vi "Host_FastOsziTest.vi"() -> ()   [LabVIEW 2012]
uses:
  <vilib>/Analysis/baseanly.llb/Mean (DBL).vi
  <vilib>/FPGAPlugInAG/PXIe-7962R/niLvFpga_Open_PXIe-7962R.vi
  <vilib>/rvi/interface/common/dynamic/niFpgaDynamicAddResources.vi
  <vilib>/Utility/error.llb/Error Cluster From Error Code.vi
  <vilib>/rvi/errors/niLvFpgaAdjustHostInterfaceError.vi
  <vilib>/FPGAPlugInAG/Dynamic/niLvFpga_Close_Dynamic.vi
  <vilib>/rvi/interface/nirviOpenFPGA/nirviOpenFPGA.xnode
  FPGA Bitfiles/NiFpga_AnalogDemultiplexerV2_NI5771.lvbitx
  <vilib>/rvi/interface/nirviReadWriteControl/nirviReadWriteControl.xnode
  <vilib>/rvi/interface/nirviMethod/nirviMethod.xnode
  <vilib>/rvi/interface/nirviCloseFPGA/nirviCloseFPGA.xnode
  <vilib>/rvi/interface/Simulation/niFpgaSimulationCallBeginRW.vi
  <vilib>/FPGAPlugInAG/Dynamic/niLvFpga_ReadFifo_Dynamic.vi
  <vilib>/rvi/errors/niLvFpgaMergeErrorWithErrorCode.vi
  <vilib>/Analysis/NI_AALPro.lvlib
  <vilib>/Analysis/NI_AALBase.lvlib
  NiFpgaLv.dll
panel:
  out "NOT Crosstalk":dbl format="%0.2f"
  out "Crosstalk":dbl format="%0.2f"
  in  "Save?":bool
  out "time to draw(ms) 2":i32=1000
  out "Area 1":picture
  in  "stop 2":bool
  in  "sized scatter plot cosmetics 2":T1={"min size"=1, "max size"=5, "maps to max size"=5, "color array"=[16711680, 65280, 255, 16776960, 16737792, 65535]}
  in  "cartesian axis attributes 2":T2={"x minimum"=1.0, "x maximum"=500.0, "x log?"=FALSE, "x precision"=1, "x format"=enum."Decimal", "y minimum"=60.0, "y maximum"=740.0, "y log?"=FALSE, "y precision"=1, "y format"=enum."Decimal"} {"x minimum" format="%0.2f"; "x maximum" format="%0.2f"; "y minimum" format="%0.2f"; "y maximum" format="%0.2f"}
  in  "?":u16(ring)=4 items=["Points", "Squares", "Circles", "Sized Squares", "Sized-Colored Squares", "Min-Max Lines"]
  in  "line color 2":u32(colorbox)=39168
  in  "text color 2":u32(colorbox)=65280
  in  "plot color 2":u32(colorbox)=16776960
  out "time to draw(ms)":i32=1000
  out "Area 2":picture
  in  "stop":bool
  in  "sized scatter plot cosmetics":T1={"min size"=1, "max size"=5, "maps to max size"=5, "color array"=[16711680, 65280, 255, 16776960, 16737792, 65535]}
  in  "cartesian axis attributes":T2={"x minimum"=1.0, "x maximum"=500.0, "x log?"=FALSE, "x precision"=1, "x format"=enum."Decimal", "y minimum"=60.0, "y maximum"=740.0, "y log?"=FALSE, "y precision"=1, "y format"=enum."Decimal"} {"x minimum" format="%0.2f"; "x maximum" format="%0.2f"; "y minimum" format="%0.2f"; "y maximum" format="%0.2f"}
  in  "?":u16(ring)=4 items=["Points", "Squares", "Circles", "Sized Squares", "Sized-Colored Squares", "Min-Max Lines"]
  in  "line color":u32(colorbox)=39168
  in  "text color":u32(colorbox)=65280
  in  "plot color":u32(colorbox)=16776960
  out "PMT histogram":T3(graph)
  out "Mean NOT pulse length":dbl format="%0.2f"
  out "Mean pulse length":dbl format="%0.2f"
  out "NOT Laser pulse length histogram":T3(graph)
  out "Laser pulse length histogram":T3(graph)
  out "Laser (Trigger In)":i16[](graph)
  in  "Samples per pixel":u32=10000
  out "IO Module\\AI Over Range":bool
  out "PMT (AI 0)":u8[](graph)
  # "Sampling at 1.5GHz => 0.66 ns sampling interval"
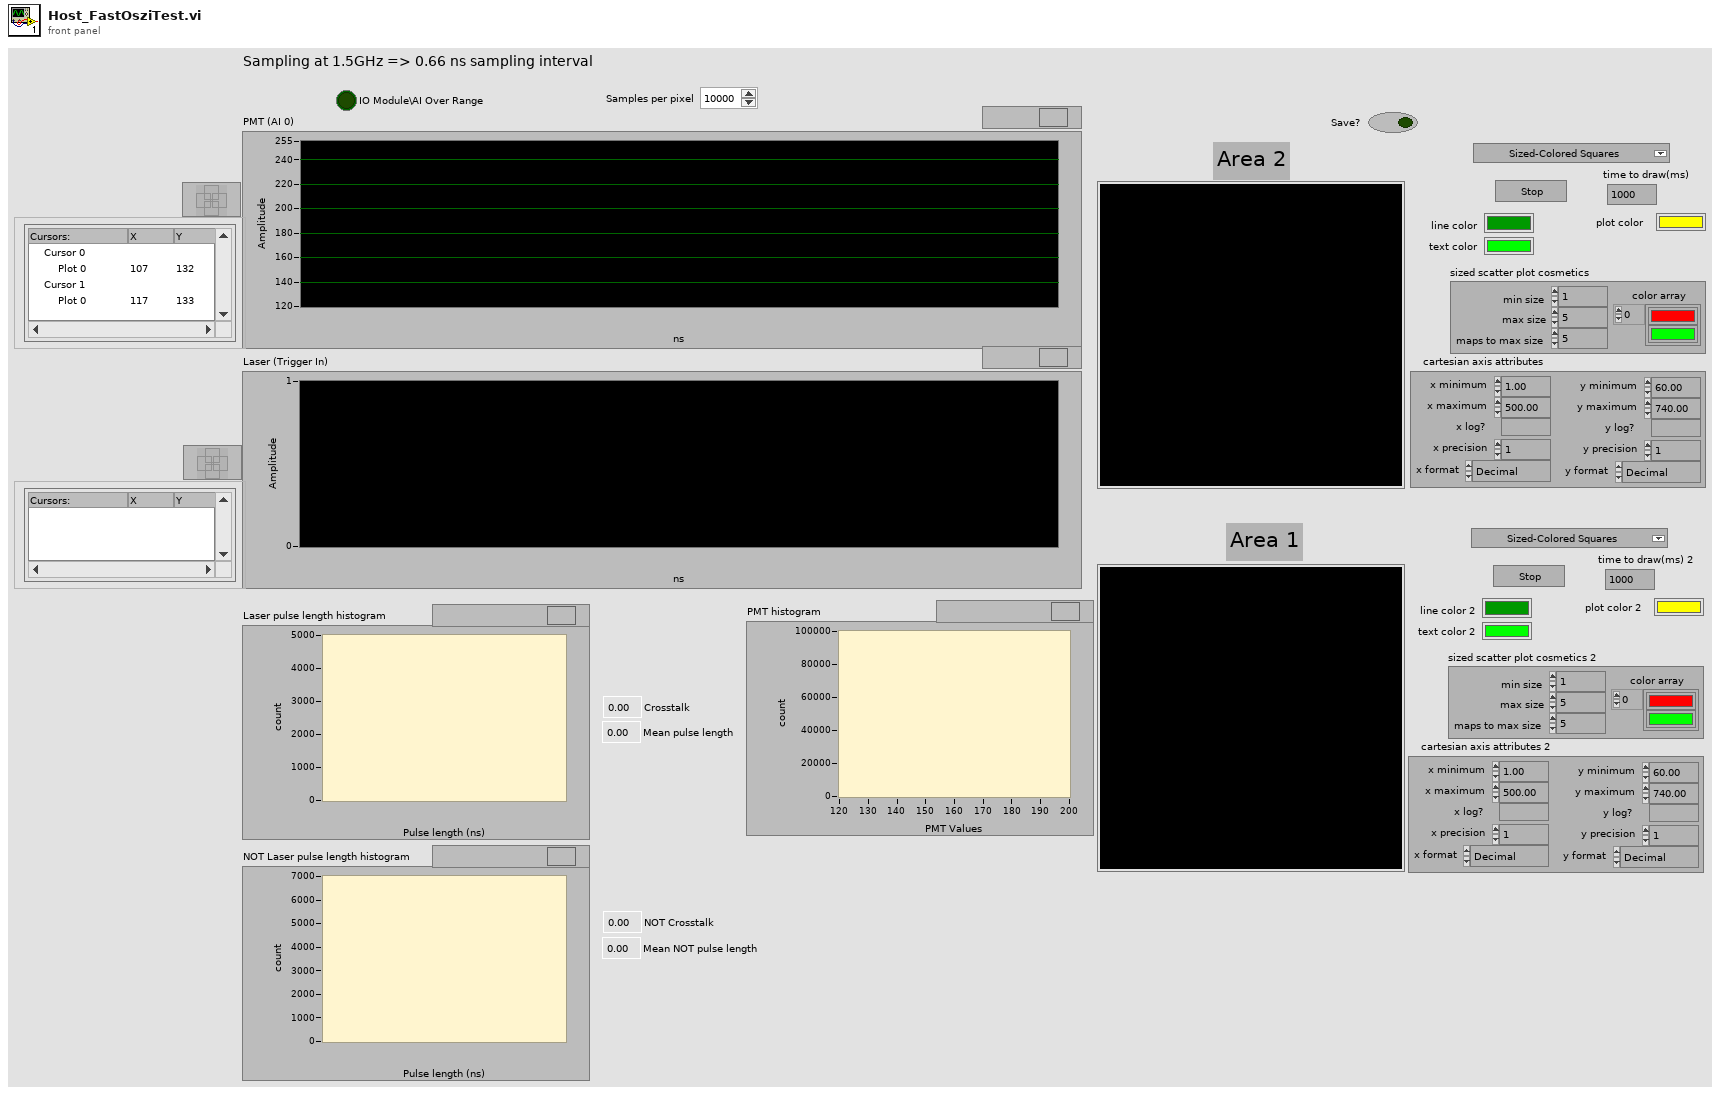
[diagram p1: front panel]
types:
  T1 = cluster{"min size":i16, "max size":i16, "maps to max size":i16, "color array":u32[]}
  T2 = cluster{"x minimum":dbl, "x maximum":dbl, "x log?":bool, "x precision":u8, "x format":enum8{"Decimal", "Scientific", "Engineering", "Binary", "Octal", "Hex"}, "y minimum":dbl, "y maximum":dbl, "y log?":bool, "y precision":u8, "y format":enum8{"Decimal", "Scientific", "Engineering", "Binary", "Octal", "Hex"}}
  T3 = cluster{"X Values":dbl[], "Histogram: h(x)":i32[]}
  T4 = cluster{"line color 2":u32, "text color 2":u32, "tick length":i16, "not crossing axes":bool, "no grids":bool}
  T5 = cluster{"plot color 2":u32, i32, "baseline(not used for these plots)":i16}
  T6 = typedef "LVBoundsTypeDef.ctl" = cluster{"Width":u32, "Height":u32}
  T7 = cluster{cluster{i32, i32, "Width":u32, "Height":u32}, "cartesian axis attributes 2":cluster{"x minimum":dbl, "x maximum":dbl, "x log?":bool, "x precision":u8, "x format":enum8{"Decimal", "Scientific", "Engineering", "Binary", "Octal", "Hex"}, "y minimum":dbl, "y maximum":dbl, "y log?":bool, "y precision":u8, "y format":enum8{"Decimal", "Scientific", "Engineering", "Binary", "Octal", "Hex"}}, cluster{"line color 2":u32, "text color 2":u32, "tick length":i16, "not crossing axes":bool, "no grids":bool}, cluster{"plot color 2":u32, i32, "baseline(not used for these plots)":i16}, "sized scatter plot cosmetics 2":cluster{"min size":i16, "max size":i16, "maps to max size":i16, "color array":u32[]}}
  T8 = cluster{"line color":u32, "text color":u32, "tick length":i16, "not crossing axes":bool, "no grids":bool}
  T9 = cluster{"plot color":u32, i32, "baseline(not used for these plots)":i16}
  T10 = cluster{cluster{i32, i32, "Width":u32, "Height":u32}, "cartesian axis attributes":cluster{"x minimum":dbl, "x maximum":dbl, "x log?":bool, "x precision":u8, "x format":enum8{"Decimal", "Scientific", "Engineering", "Binary", "Octal", "Hex"}, "y minimum":dbl, "y maximum":dbl, "y log?":bool, "y precision":u8, "y format":enum8{"Decimal", "Scientific", "Engineering", "Binary", "Octal", "Hex"}}, cluster{"line color":u32, "text color":u32, "tick length":i16, "not crossing axes":bool, "no grids":bool}, cluster{"plot color":u32, i32, "baseline(not used for these plots)":i16}, "sized scatter plot cosmetics":cluster{"min size":i16, "max size":i16, "maps to max size":i16, "color array":u32[]}}
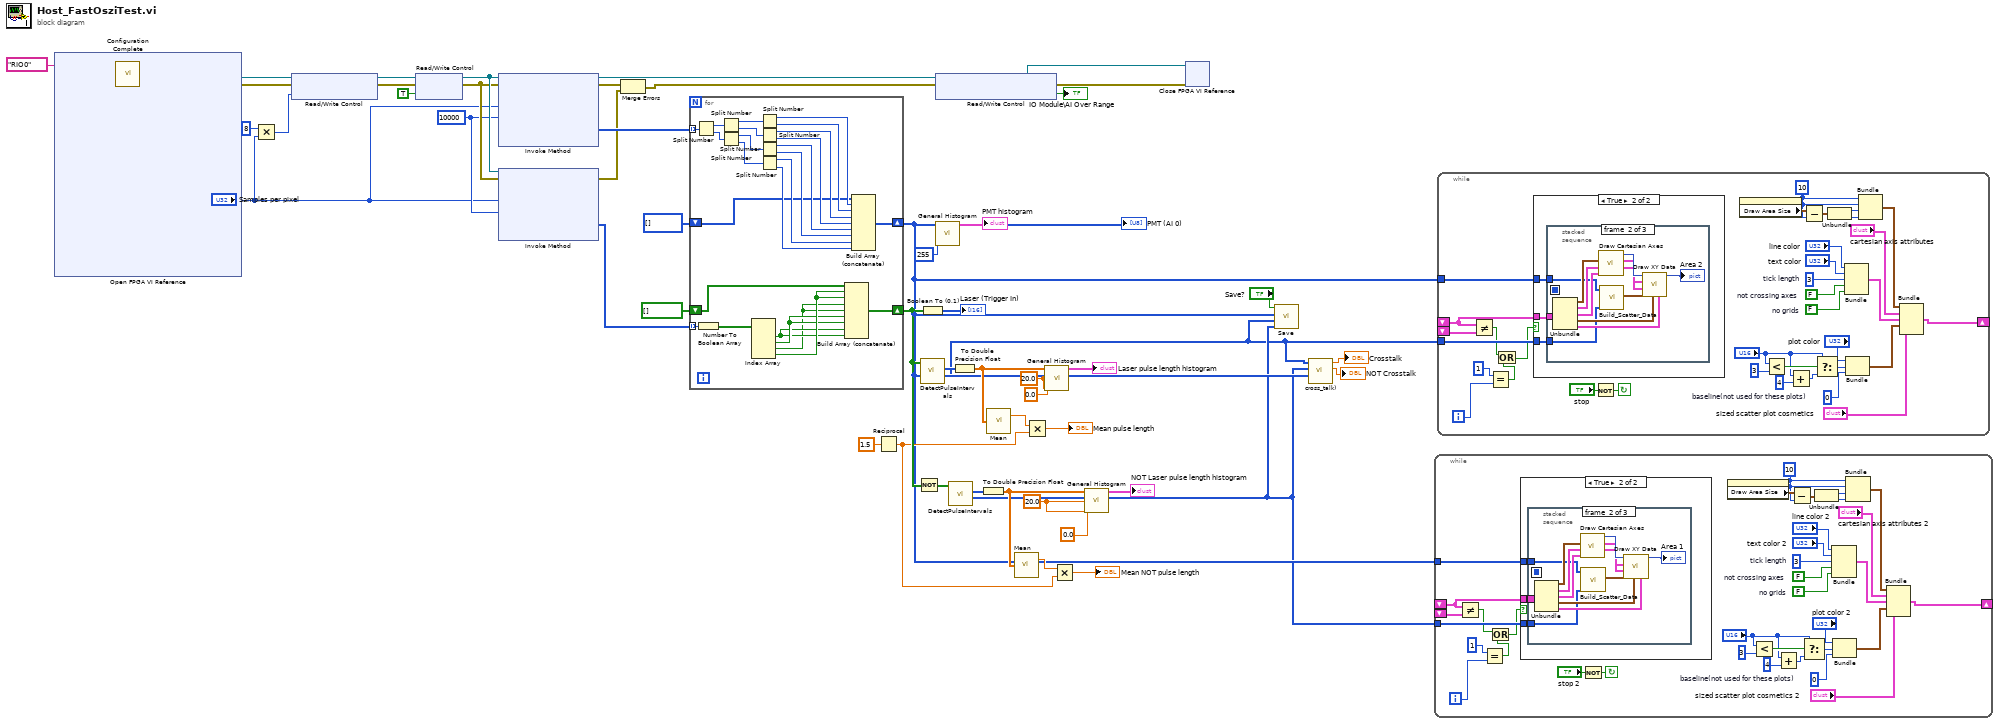
[diagram p0: block diagram]
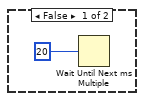
[diagram p2: hidden frame]
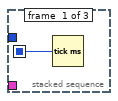
[diagram p3: hidden frame]
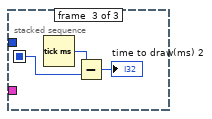
[diagram p4: hidden frame]
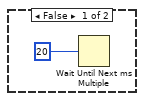
[diagram p5: hidden frame]
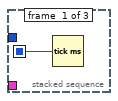
[diagram p6: hidden frame]
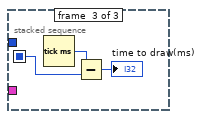
[diagram p7: hidden frame]
diagram:
  w21 = 20.0 ("max")
  w20 = 20.0 ("max")
  w33 = 10000 ("Timeout (ms)")
  n1 = xnode "Open FPGA VI Reference"("resource name"=tag "RIO0") -> ("FPGA VI Reference Out"=w1:refnum<k20>, "error out"=w51:errorcluster)  [unwired: 1 in]
  n2 = call "Configuration Complete.vi"("error in"=w51, "FPGA VI Reference In"=w1) -> ("error out"=w49:errorcluster, "FPGA VI Reference Out"=w50:refnum<k20>)  [unwired: 7 in, 1 out]
  n3 = Multiply(x=u32 8, y="Samples per pixel") -> (x*y=w40:u32)
  n4 = xnode "Read/Write Control"("FPGA VI Reference In"=w50, "error in"=w49, "Samples per pixel"=w40) -> ("FPGA VI Reference Out"=w47:refnum<k20>, "error out"=w48:errorcluster)
  n5 = xnode "Read/Write Control"("FPGA VI Reference In"=w47, "error in"=w48, "Acquire"=TRUE) -> ("FPGA VI Reference Out"=w38:refnum<k20>, "error out"=w37:errorcluster)
  n6 = xnode "Invoke Method"("FPGA VI Reference In"=w38, "error in"=w37, "Number of Elements"="Samples per pixel", "Timeout (ms)"=w33) -> ("FPGA VI Reference Out"=w45:refnum<k20>, "error out"=w36:errorcluster, "Data"=w39:u64[])  [unwired: 1 out]
  n7 = xnode "Invoke Method"("FPGA VI Reference In"=w38, "error in"=w37, "Number of Elements"="Samples per pixel", "Timeout (ms)"=w33) -> ("error out"=w34:errorcluster, "Data"=w31:u64[])  [unwired: 2 out]
  n8 = Merge Errors(w36, w34) -> (w35:errorcluster)
  n9 = for {
    tunnel: w39 -> [w77] mode=indexing
    shift-right: [w62] -> w6
    shift-left: u8[] [] -> [w61]
    tunnel: w31 -> [w60] mode=indexing
    shift-right: [w55] -> w27
    shift-left: bool[] [] -> [w54]
    n10 = Split Number(x=w77) -> (hi(x)=w76:u32, lo(x)=w75:u32)
    n11 = Number To Boolean Array(number=w60) -> (Boolean array=w53:bool[])
    n12 = Split Number(x=w76) -> (hi(x)=w74:u16, lo(x)=w73:u16)
    n13 = Split Number(x=w75) -> (hi(x)=w72:u16, lo(x)=w71:u16)
    n14 = Index Array(array=w53) -> (element #1=w57:bool, element #2=w58:bool, element #3=w56:bool, element #4=w59:bool)  [unwired: 4 in]
    n15 = Split Number(x=w74) -> (hi(x)=w70:u8, lo(x)=w69:u8)
    n16 = Split Number(x=w73) -> (hi(x)=w68:u8, lo(x)=w67:u8)
    n17 = Split Number(x=w72) -> (hi(x)=w66:u8, lo(x)=w65:u8)
    n18 = Split Number(x=w71) -> (hi(x)=w64:u8, lo(x)=w63:u8)
    n19 = Build Array (concatenate)(w54, w59, w59, w56, w56, w58, w58, w57, w57) -> (w55:bool[])
    n20 = Build Array (concatenate)(w61, w70, w69, w68, w67, w66, w65, w64, w63) -> (w62:u8[])
  }
  "PMT (AI 0)" <- w6
  n21 = Reciprocal(x=1.5) -> (1/x=w13:dbl)
  n22 = Not(x=w27) -> (.not. x?=w23:bool[])
  n23 = Boolean To (0,1)(Boolean=w27) -> (0, 1=→"Laser (Trigger In)":i16[])
  n24 = call "DetectPulseIntervals.vi"("Binary array probe"=w27) -> ("Rising Index"=w2:i32[], "Pulse lenghts out"=w9:i32[])  [unwired: 6 in, 3 out]
  n25 = xnode "Read/Write Control"("FPGA VI Reference In"=w45, "error in"=w35) -> ("FPGA VI Reference Out"=w44:refnum<k20>, "error out"=w43:errorcluster, "IO Module\\AI Over Range"=→"IO Module\\AI Over Range":bool)
  n26 = call <vilib>:"General Histogram.vi"("X"=w6, "# bins"=255) -> ("Histogram Graph"=→"PMT histogram":T3)  [unwired: 9 in, 4 out]
  n27 = call "DetectPulseIntervals.vi"("Binary array probe"=w23) -> ("Rising Index"=w3:i32[], "Pulse lenghts out"=w8:i32[])  [unwired: 6 in, 3 out]
  n28 = To Double Precision Float(number=w9) -> (double precision float=w19:dbl[])
  n29 = To Double Precision Float(number=w8) -> (double precision float=w12:dbl[])
  n30 = call-poly <vilib>:"Mean.vi"("X"=w19) -> ("mean"=w17:dbl)  [unwired: 1 out]
  n31 = call-poly <vilib>:"Mean.vi"("X"=w12) -> ("mean"=w14:dbl)  [unwired: 1 out]
  n32 = Multiply(x=w17, y=w13) -> (x*y=→"Mean pulse length":dbl)
  n33 = call <vilib>:"General Histogram.vi"("X"=w19, "max"=w20, "min"=0.0, "# bins"=w20) -> ("Histogram Graph"=→"Laser pulse length histogram":T3)  [unwired: 7 in, 4 out]
  n34 = Multiply(x=w14, y=w13) -> (x*y=→"Mean NOT pulse length":dbl)
  n35 = call <vilib>:"General Histogram.vi"("X"=w12, "max"=w21, "min"=0.0, "# bins"=w21) -> ("Histogram Graph"=→"NOT Laser pulse length histogram":T3)  [unwired: 7 in, 4 out]
  n36 = xnode "Close FPGA VI Reference"("FPGA VI Reference In"=w44, "error in"=w43) -> ()  [unwired: 1 out]
  n37 = call "Save.vi"("Rising Index 1"=w3, "Rising Index 2"=w2, "PMT (AI 0)"=w6, "Save?"="Save?") -> ()  [unwired: 8 in]
  n38 = call "cross_talk).vi"("Array"=w6, "Rising Index 2"=w3, "Rising Index"=w2) -> ("x/y 2"=→"NOT Crosstalk":dbl, "x/y"=→"Crosstalk":dbl)  [unwired: 7 in]
  n39 = while {
    shift-left: _ -> [w86]
    shift-left: _ -> [w85]
    shift-right: [w87] -> _
    tunnel: w6 -> [w84]
    tunnel: w3 -> [w83]
    i -> [w81]
    stop <- w111 continue-if-true
    w95 = i16 0  # baseline(not used for these plots)
    w102 = FALSE  # not crossing axes
    w103 = i16 3  # tick length
    w101 = FALSE  # no grids
    w106 = 10
    n40 = Not Equal?(x=w85, y=w86) -> (x != y?=w80:bool)
    n41 = Equal?(x=1, y=w81) -> (x = y?=w79:bool)
    n42 = Or(x=w80, y=w79) -> (x .or. y?=w78:bool)
    n43 = case shown="True" w78 {
      tunnel: w85 -> [_ w116]
      tunnel: w84 -> [_ w115]
      tunnel: w83 -> [_ w114]
      frame False {
        n44 = Wait Until Next ms Multiple(millisecond multiple=20) -> ()  [unwired: 1 out]
      }
      frame True {
        n45 = stacked-sequence {
          seq-local: [w117 _ _] -> [_ _ w132]
          tunnel: w116 -> [_ w124 _]
          tunnel: w115 -> [_ w119 _]
          tunnel: w114 -> [_ w118 _]
          frame #0 {
            n46 = Tick Count (ms)() -> (millisecond timer value=w117:u32)
          }
          frame #1 {
            n47 = Unbundle(w124) -> (w125:cluster{i32, i32, "Width":u32, "Height":u32}, "cartesian axis attributes 2"=w126:T2, w127:T4, w122:T5, "sized scatter plot cosmetics 2"=w121:T1)
            n48 = call <vilib>:"Draw Cartesian Axes.vi"("grid cosmetics"=w127, "axis attributes"=w126, "bounding rect"=w125) -> ("y scale factors"=w129:cluster{"a":dbl, "b":dbl, "log?":bool}, "x scale factors"=w128:cluster{"a":dbl, "b":dbl, "log?":bool}, "new picture"=w130:picture)  [unwired: 6 in]
            n49 = call "Build_Scatter_Data.vi"("Rising Index"=w118, "PMT (AI 0)"=w119) -> ("data"=w120:cluster{"x":dbl, "y":dbl}[])  [unwired: 9 in]
            n50 = call <vilib>:"Draw XY Data.vi"("[sized scatter plot cosmetics]"=w121, "xy cosmetics"=w122, "xy data"=w120, "y scale factors"=w129, "x scale factors"=w128, "picture"=w130) -> ("new picture"=→"Area 1":picture)  [unwired: 5 in]
          }
          frame #2 {
            n51 = Tick Count (ms)() -> (millisecond timer value=w133:u32)
            n52 = Subtract(x=w133, y=w132) -> (x-y=→"time to draw(ms) 2":u32)
          }
        }
      }
    }
    n53 = Not(x="stop 2") -> (.not. x?=w111:bool)
    n54 = property on="Area 1" class="Pict"() -> ("Draw Area Size"=w110:T6)  [unwired: 2 in, 2 out]
    n55 = Less?(x="?", y=3) -> (x < y?=w100:bool)
    n56 = Add(x="?", y=4) -> (x+y=w98:i32)
    n57 = Subtract(x=w110, y=w106) -> (x-y=w109:T6)
    n58 = Select(t="?", s=w100, f=w98) -> (s? t:f=w96:i32)
    n59 = Unbundle(w109) -> ("Width"=w107:u32, "Height"=w108:u32)
    n60 = Bundle("line color 2"="line color 2", "text color 2"="text color 2", "tick length"=w103, "not crossing axes"=w102, "no grids"=w101) -> (w90:T4)  [unwired: 1 in]
    n61 = Bundle("plot color 2"="plot color 2", w96, "baseline(not used for these plots)"=w95) -> (w91:T5)  [unwired: 1 in]
    n62 = Bundle(w106, w106, "Width"=w107, "Height"=w108) -> (w88:cluster{i32, i32, "Width":u32, "Height":u32})  [unwired: 1 in]
    n63 = Bundle(w88, "cartesian axis attributes 2"="cartesian axis attributes 2", w90, w91, "sized scatter plot cosmetics 2"="sized scatter plot cosmetics 2") -> (w87:T7)  [unwired: 1 in]
  }
  n64 = while {
    shift-left: _ -> [w142]
    shift-left: _ -> [w141]
    shift-right: [w143] -> _
    tunnel: w6 -> [w140]
    tunnel: w2 -> [w139]
    i -> [w136]
    stop <- w167 continue-if-true
    w151 = i16 0  # baseline(not used for these plots)
    w158 = FALSE  # not crossing axes
    w159 = i16 3  # tick length
    w157 = FALSE  # no grids
    w162 = 10
    n65 = Not Equal?(x=w141, y=w142) -> (x != y?=w135:bool)
    n66 = Equal?(x=1, y=w136) -> (x = y?=w137:bool)
    n67 = Or(x=w135, y=w137) -> (x .or. y?=w134:bool)
    n68 = case shown="True" w134 {
      tunnel: w141 -> [_ w172]
      tunnel: w140 -> [_ w171]
      tunnel: w139 -> [_ w170]
      frame False {
        n69 = Wait Until Next ms Multiple(millisecond multiple=20) -> ()  [unwired: 1 out]
      }
      frame True {
        n70 = stacked-sequence {
          seq-local: [w173 _ _] -> [_ _ w188]
          tunnel: w172 -> [_ w180 _]
          tunnel: w171 -> [_ w175 _]
          tunnel: w170 -> [_ w174 _]
          frame #0 {
            n71 = Tick Count (ms)() -> (millisecond timer value=w173:u32)
          }
          frame #1 {
            n72 = Unbundle(w180) -> (w181:cluster{i32, i32, "Width":u32, "Height":u32}, "cartesian axis attributes"=w182:T2, w183:T8, w178:T9, "sized scatter plot cosmetics"=w177:T1)
            n73 = call <vilib>:"Draw Cartesian Axes.vi"("grid cosmetics"=w183, "axis attributes"=w182, "bounding rect"=w181) -> ("y scale factors"=w185:cluster{"a":dbl, "b":dbl, "log?":bool}, "x scale factors"=w184:cluster{"a":dbl, "b":dbl, "log?":bool}, "new picture"=w186:picture)  [unwired: 6 in]
            n74 = call "Build_Scatter_Data.vi"("Rising Index"=w174, "PMT (AI 0)"=w175) -> ("data"=w176:cluster{"x":dbl, "y":dbl}[])  [unwired: 9 in]
            n75 = call <vilib>:"Draw XY Data.vi"("[sized scatter plot cosmetics]"=w177, "xy cosmetics"=w178, "xy data"=w176, "y scale factors"=w185, "x scale factors"=w184, "picture"=w186) -> ("new picture"=→"Area 2":picture)  [unwired: 5 in]
          }
          frame #2 {
            n76 = Tick Count (ms)() -> (millisecond timer value=w189:u32)
            n77 = Subtract(x=w189, y=w188) -> (x-y=→"time to draw(ms)":u32)
          }
        }
      }
    }
    n78 = Not(x="stop") -> (.not. x?=w167:bool)
    n79 = property on="Area 2" class="Pict"() -> ("Draw Area Size"=w166:T6)  [unwired: 2 in, 2 out]
    n80 = Less?(x="?", y=3) -> (x < y?=w156:bool)
    n81 = Add(x="?", y=4) -> (x+y=w154:i32)
    n82 = Subtract(x=w166, y=w162) -> (x-y=w165:T6)
    n83 = Select(t="?", s=w156, f=w154) -> (s? t:f=w152:i32)
    n84 = Unbundle(w165) -> ("Width"=w163:u32, "Height"=w164:u32)
    n85 = Bundle("line color"="line color", "text color"="text color", "tick length"=w159, "not crossing axes"=w158, "no grids"=w157) -> (w146:T8)  [unwired: 1 in]
    n86 = Bundle("plot color"="plot color", w152, "baseline(not used for these plots)"=w151) -> (w147:T9)  [unwired: 1 in]
    n87 = Bundle(w162, w162, "Width"=w163, "Height"=w164) -> (w144:cluster{i32, i32, "Width":u32, "Height":u32})  [unwired: 1 in]
    n88 = Bundle(w144, "cartesian axis attributes"="cartesian axis attributes", w146, w147, "sized scatter plot cosmetics"="sized scatter plot cosmetics") -> (w143:T10)  [unwired: 1 in]
  }
